vi "Read Voltage Datas.vi"(8 "error in (no error)":errorcluster, 9 "length":u32, 10 "buffer":dbl[](array[numeric])=array[1048576 elements], 11 "channel":i8) -> (0 "error out":errorcluster, 2 "buffer out":dbl[](array[numeric]), 3 "function return":u32)   [LabVIEW 2021, in "vmmsolib.lvlib"]
doc: "DLL_API unsigned int WINAPI ReadVoltageDatas(char channel, double* buffer, unsigned int length);"
uses:
  vmmsolib.lvlib
  vmmso.dll
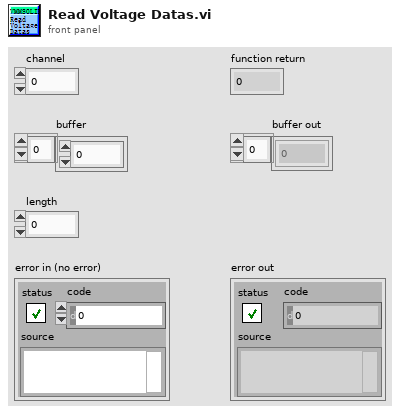
[diagram p1: front panel]
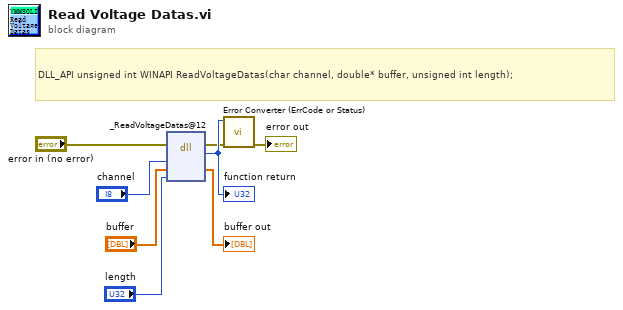
[diagram p0: block diagram]
diagram:
  # "DLL_API unsigned int WINAPI ReadVoltageDatas(char channel, double* buffer, unsigned int length);"
  n1 = dll-call lib="D:/VmMsoSDK/demo-Labview/2021/vmmsolib/vmmso.*" fn="_ReadVoltageDatas@12"(error in="error in (no error)", "channel"="channel", "buffer"="buffer", "length"="length") -> (error out=w2:errorcluster, w8:u32, "buffer"=→"buffer out":dbl[])  [unwired: 4 in, 1 out]
  "function return" <- w8
  n2 = call "Error Converter (ErrCode or Status).vi"("error in (no error)"=w2, "error code"=w8) -> ("error out"=→"error out":errorcluster)  [unwired: 9 in]
